vi "CableMotorSensorMismatch.vi"(1 "Conversion":T1, 3 "Input":dbl[](array[numeric])) -> (0 "Output":dbl[](array[numeric]))   [LabVIEW 2015]
uses:
  <userlib>/_OpenG.lib/array/array.llb/Index 1D Array Elements (DBL)__ogtk.vi
panel:
  out "SensorID":i32[](array[numeric])
  out "MotorID":i32[](array[numeric])
  out "CableID":i32[](array[numeric])
  out "Sensor0":dbl[](array[numeric])
  out "Motor0":dbl[](array[numeric])
  out "Cable0":dbl[](array[numeric])
  in  "Cconversion Table":T2(array[cluster])=[{"CableID"=4, "MotorID"=8, "SensorID"=8, "Total"=TRUE}, {"CableID"=1, "MotorID"=1, "SensorID"=5, "Total"=FALSE}, {"CableID"=3, "MotorID"=2, "SensorID"=6, "Total"=FALSE}, {"CableID"=4, "MotorID"=3, "SensorID"=7, "Total"=FALSE}, {"CableID"=2, "MotorID"=4, "SensorID"=8, "Total"=FALSE}]
  # "Total number of Cable/Motor/Sensor"
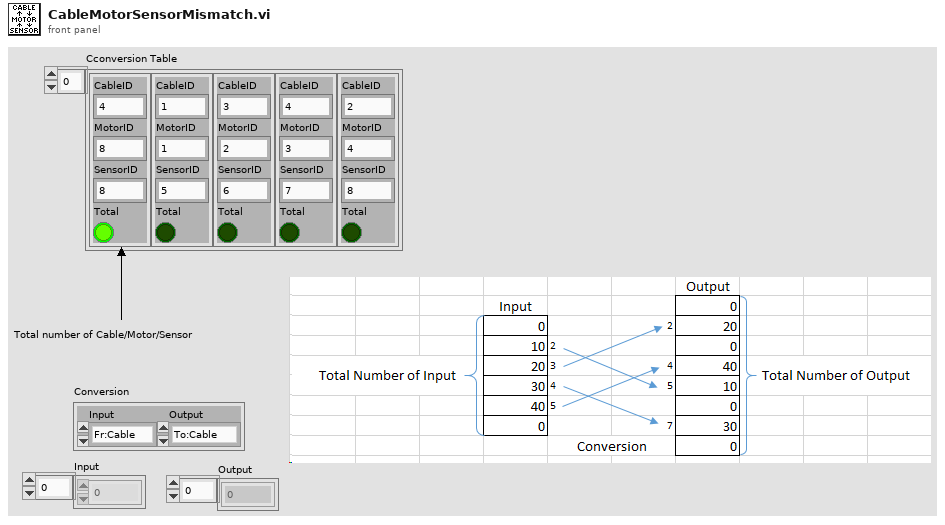
[diagram p1: front panel]
types:
  T1 = cluster{"Input":enum16{"Fr:Cable", "Fr:Motor", "Fr:Sensor"}, "Output":enum16{"To:Cable", "To:Motor", "To:Sensor"}}
  T2 = cluster{"CableID":i32, "MotorID":i32, "SensorID":i32, "Total":bool}[]
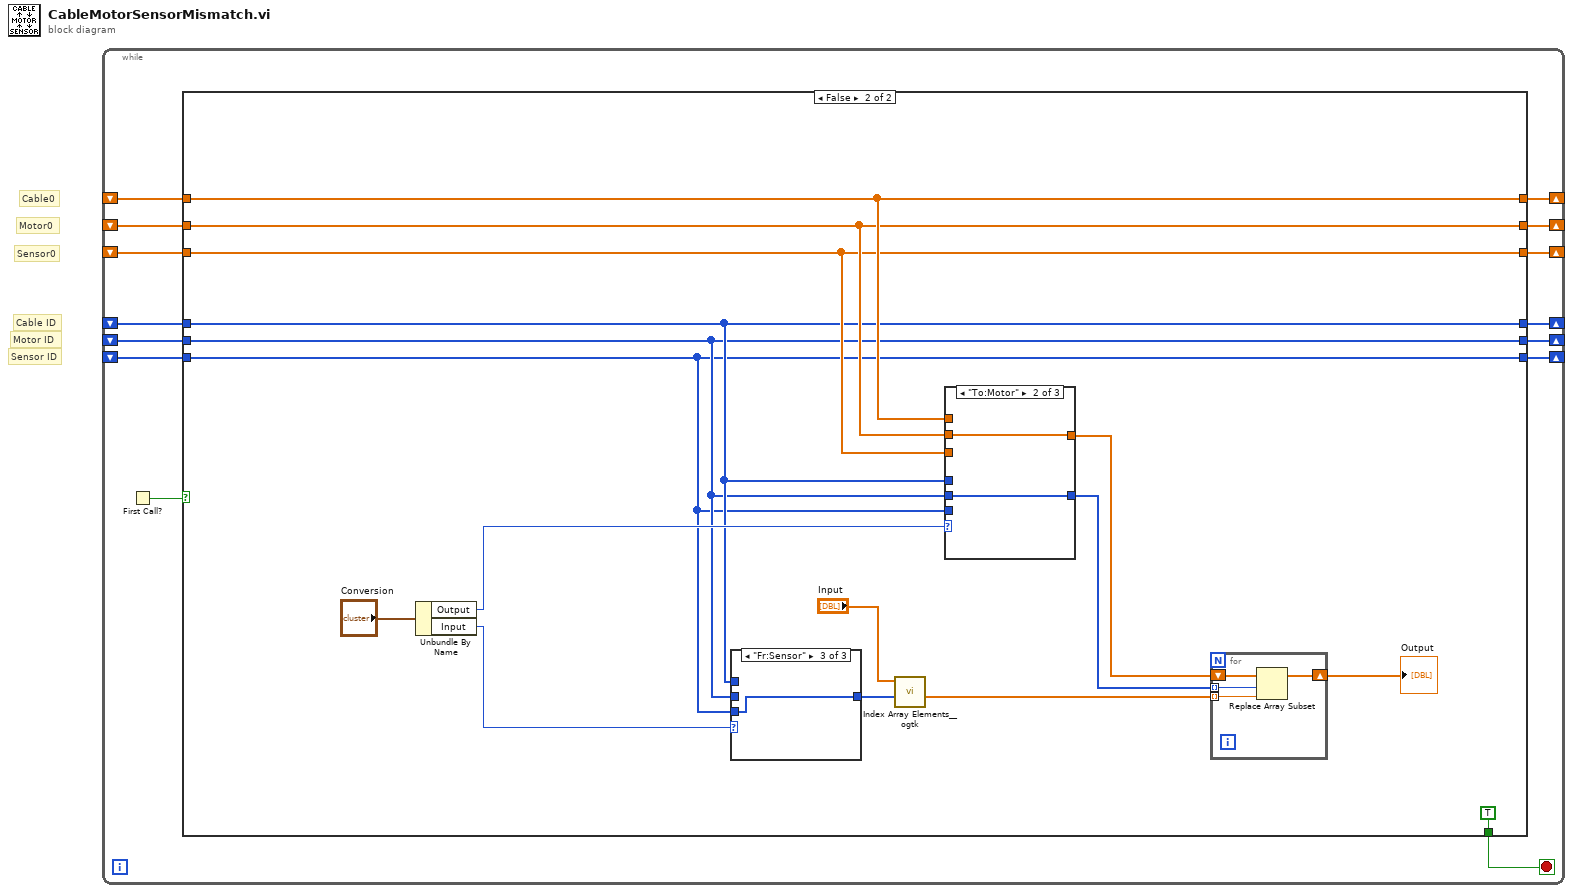
[diagram p0: block diagram]
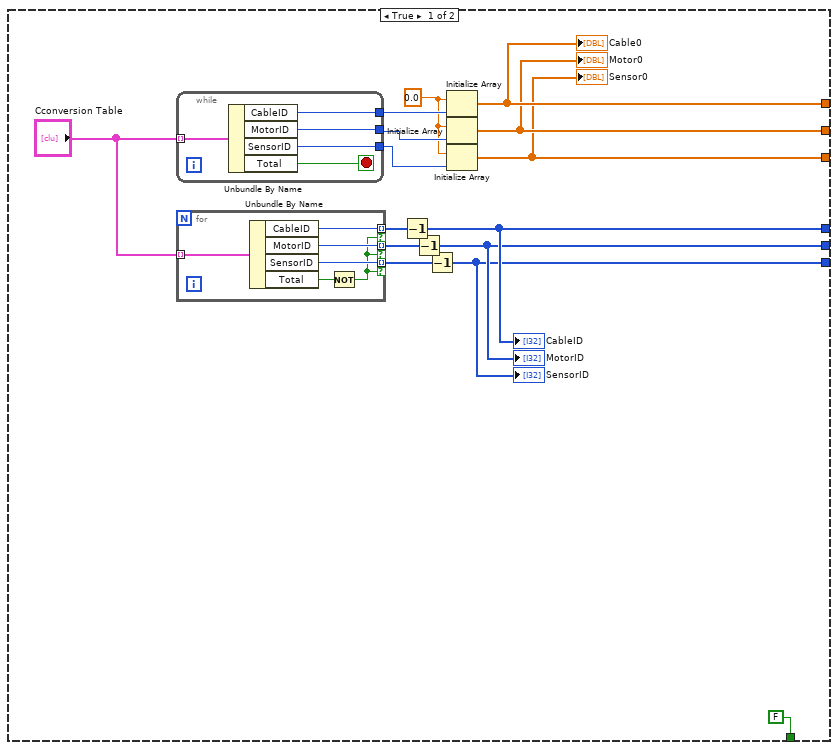
[diagram p2: hidden frame]
diagram:
  # "Sensor ID"
  # "Motor ID"
  # "Cable ID"
  # "Sensor0"
  # "Motor0"
  # "Cable0"
  n1 = while {
    shift-right: [w14] -> _
    shift-left: _ -> [w8]
    shift-right: [w13] -> _
    shift-left: _ -> [w7]
    shift-right: [w12] -> _
    shift-left: _ -> [w6]
    shift-right: [w11] -> _
    shift-left: _ -> [w5]
    shift-right: [w10] -> _
    shift-left: _ -> [w4]
    shift-right: [w9] -> _
    shift-left: _ -> [w3]
    stop <- w2 stop-if-true
    n2 = First Call?() -> (First Call?: T/F=w1:bool)
    n3 = case shown="False" w1 {
      tunnel: [w28 w50] -> w14
      tunnel: [w27 w49] -> w13
      tunnel: [w26 w48] -> w12
      tunnel: [w25 w47] -> w11
      tunnel: [w24 w46] -> w10
      tunnel: [w23 w45] -> w9
      tunnel: w8 -> [_ w50]
      tunnel: w7 -> [_ w49]
      tunnel: w6 -> [_ w48]
      tunnel: w5 -> [_ w47]
      tunnel: w4 -> [_ w46]
      tunnel: w3 -> [_ w45]
      tunnel: [FALSE TRUE] -> w2
      frame True {
        w19 = 0.0 ("element")
        n4 = while {
          tunnel: "Cconversion Table" -> [w40] mode=indexing
          tunnel: [w38] -> w22
          tunnel: [w37] -> w21
          tunnel: [w36] -> w20
          stop <- w39 stop-if-true
          n5 = Unbundle By Name(w40) -> ("CableID"=w38:i32, "MotorID"=w37:i32, "SensorID"=w36:i32, "Total"=w39:bool)
        }
        n6 = for {
          tunnel: "Cconversion Table" -> [w35] mode=indexing
          tunnel: [w34] -> w16 mode=indexing if=w30
          tunnel: [w33] -> w18 mode=indexing if=w30
          tunnel: [w32] -> w17 mode=indexing if=w30
          n7 = Unbundle By Name(w35) -> ("CableID"=w34:i32, "MotorID"=w33:i32, "SensorID"=w32:i32, "Total"=w31:bool)
          n8 = Not(x=w31) -> (.not. x?=w30:bool)
        }
        n9 = Decrement(x=w16) -> (x-1=w25:i32[])
        "CableID" <- w25
        n10 = Decrement(x=w18) -> (x-1=w24:i32[])
        "MotorID" <- w24
        n11 = Decrement(x=w17) -> (x-1=w23:i32[])
        "SensorID" <- w23
        n12 = Initialize Array(w19, w22) -> (w28:dbl[])
        "Cable0" <- w28
        n13 = Initialize Array(w19, w21) -> (w27:dbl[])
        "Motor0" <- w27
        n14 = Initialize Array(w19, w20) -> (w26:dbl[])
        "Sensor0" <- w26
      }
      frame False {
        n15 = Unbundle By Name("Conversion") -> ("Output"=w51:enum16{"To:Cable", "To:Motor", "To:Sensor"}, "Input"=w52:enum16{"Fr:Cable", "Fr:Motor", "Fr:Sensor"})
        n16 = case shown="\"Fr:Sensor\"" w52 {
          tunnel: w47 -> [w63 _ _]
          tunnel: w46 -> [_ w64 _]
          tunnel: w45 -> [_ _ w65]
          tunnel: [w63 w64 w65] -> w55
          frame "Fr:Cable" {
          }
          frame "Fr:Motor" {
          }
          frame "Fr:Sensor" {
          }
        }
        n17 = call-poly <userlib>:"Index Array Elements__ogtk.vi"("indices"=w55, "array"="Input") -> ("elements"=w56:dbl[])  [unwired: 9 in]
        n18 = case shown="\"To:Motor\"" w51 {
          tunnel: w47 -> [w58 _ _]
          tunnel: w46 -> [_ w60 _]
          tunnel: w45 -> [_ _ w62]
          tunnel: [w58 w60 w62] -> w53
          tunnel: w50 -> [w57 _ _]
          tunnel: w49 -> [_ w59 _]
          tunnel: w48 -> [_ _ w61]
          tunnel: [w57 w59 w61] -> w54
          frame "To:Cable" {
          }
          frame "To:Motor" {
          }
          frame "To:Sensor" {
          }
        }
        n19 = for {
          tunnel: w53 -> [w68] mode=indexing
          tunnel: w56 -> [w67] mode=indexing
          shift-right: [w66] -> w43
          shift-left: w54 -> [w69]
          n20 = Replace Array Subset(array=w69, new element=w67, index=w68) -> (w66:dbl[])
        }
        "Output" <- w43
      }
    }
  }
